vi "Revision Query.vi"(8 "error in (no error)":errorcluster, 11 "VISA resource name":refnum<visa-resource-name>) -> (0 "error out":errorcluster, 1 "Serial Number":string, 2 "Model":string, 3 "VISA resource name out":refnum<visa-resource-name>, 4 "Firmware Revision":string, 5 "Manufacturer":string)   [LabVIEW 2015, in "Keysight U1252.lvlib"]
doc: "Queries the current instrument firmware revision and instrument driver revision.\n\nRefer to the Readme file for detailed driver information including modification history."
uses:
  <instrlib>/Keysight U1252/Keysight U1252.lvlib
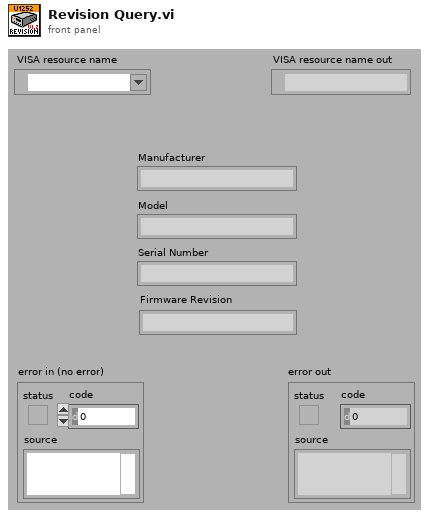
[diagram p1: front panel]
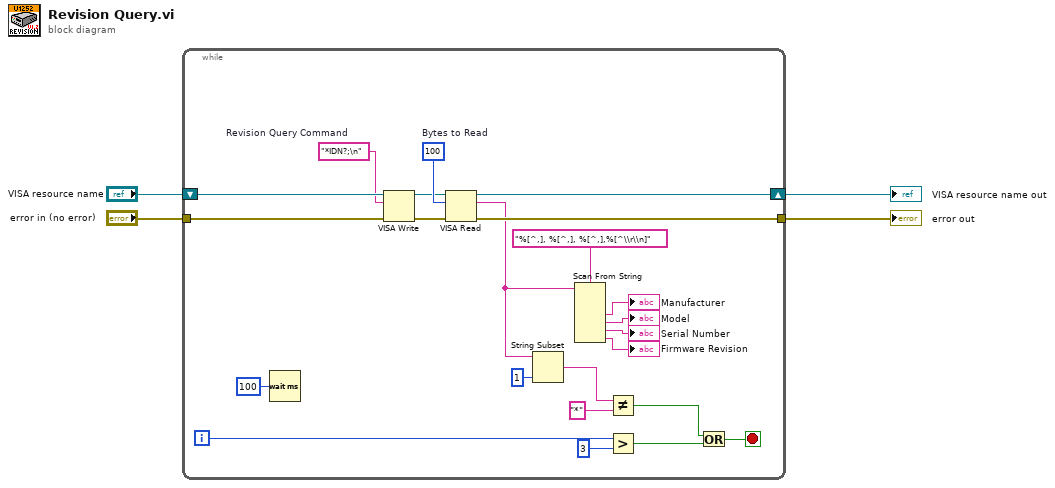
[diagram p0: block diagram]
diagram:
  n1 = while {
    shift-right: [w19] -> w2
    shift-left: "VISA resource name" -> [w27]
    tunnel: "error in (no error)" -> [w18]
    tunnel: [w20] -> w3
    i -> [w8]
    stop <- w9 stop-if-true
    w22 = "*IDN?;\n"  # Revision Query Command
    w25 = u32 100  # Bytes to Read
    n2 = Wait (ms)(milliseconds to wait=u32 100) -> ()  [unwired: 1 out]
    n3 = VISA Write(VISA resource name=w27, write buffer=w22, error in (no error)=w18) -> (VISA resource name out=w24:refnum<visa-resource-name>, error out=w23:errorcluster)  [unwired: 1 out]
    n4 = VISA Read(VISA resource name=w24, byte count=w25, error in (no error)=w23) -> (VISA resource name out=w19:refnum<visa-resource-name>, read buffer=w14:string, error out=w20:errorcluster)  [unwired: 1 out]
    n5 = String Subset(string=w14, length (rest)=1 ("length (rest)")) -> (substring=w12:string)  [unwired: 1 in]
    n6 = Scan From String(format string="%[^,], %[^,], %[^,],%[^\\r\\n]", input string=w14) -> (output 1=→"Manufacturer":string, output 2=→"Model":string, output 3=→"Serial Number":string, output 4=→"Firmware Revision":string)  [unwired: 6 in, 3 out]
    n7 = Not Equal?(x=w12, y="*") -> (x != y?=w10:bool)
    n8 = Greater?(x=w8, y=3) -> (0:w6:bool)
    n9 = Or(x=w10, y=w6) -> (x .or. y?=w9:bool)
  }
  "VISA resource name out" <- w2
  "error out" <- w3
